vi "SignalReceiver.TestLauncher.vi"() -> ()   [LabVIEW 2020, in "ECU_Diagnose.lvlib" / "SignalReceiver.lvclass"]
doc: "JKI State Machine Objects (SMO) 1.0.0.5\nJKI - JKI\nCopyright (c) 2016, JKI"
uses:
  SignalReceiver.lvclass
  <vilib>/JKI/JKI SMO/SMO/SMO.lvclass
  <vilib>/JKI/JKI SMO/SMO/Typedefs/SMOState --Enum.ctl
  GlobalData_operation.ctl
  C:/Program Files (x86)/National Instruments/LabVIEW 2020/vi.lib/JKI/JKI SMO/SMO/SMO.lvclass
  D:/BingoGithub/ECU_DiagnoseSMO_V001.06/ECU_Diagnose/SignalReceiver/SignalReceiver.lvclass
  Typedefs/Data.ctl
panel:
  out "Waveform Graph":dbl[][](graph)
  out "SignalDatOut":dbl[][](array[numeric])
  in  "StartStop":bool
  out "Value":T1
  in  "Setpoint":dbl(slide) scale=0.0..10.0
  out "error out":errorcluster
  in  "Stop":bool
  # "Timed Loop Test Launcher"
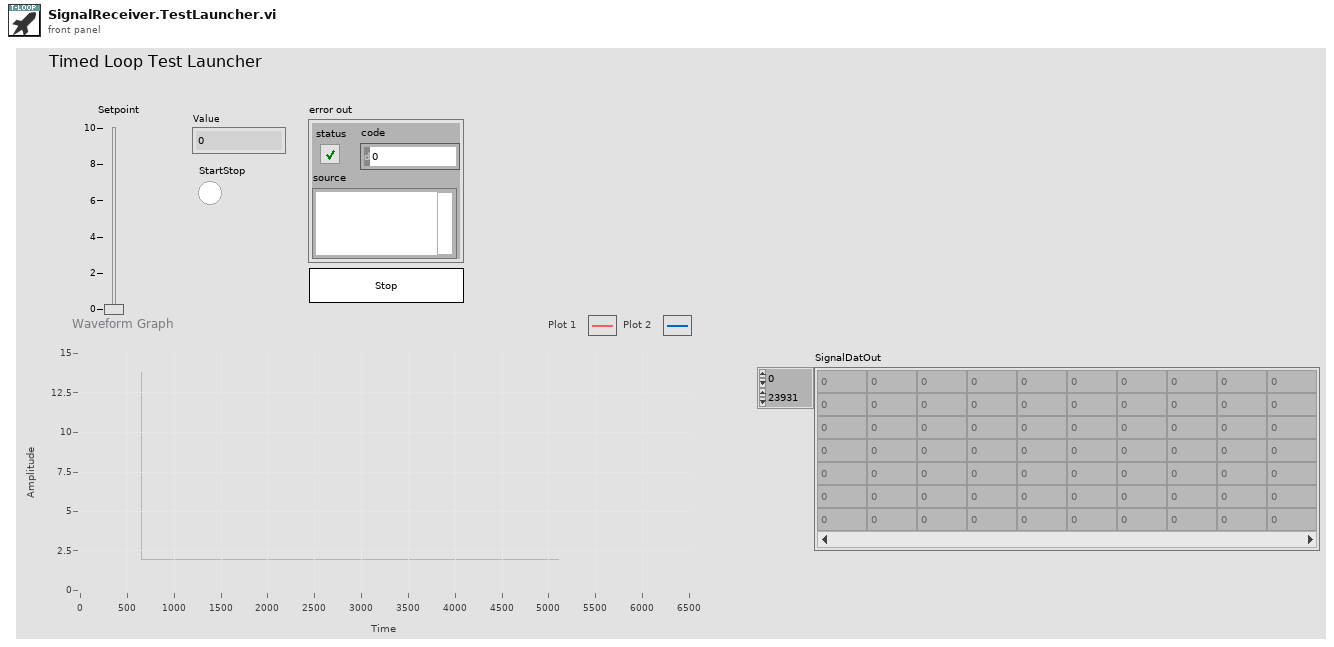
[diagram p1: front panel]
types:
  T1 = typedef "Data.ctl" = dbl
  T2 = typedef "ECU_Diagnose.lvlib/SignalReceiver.lvclass/SignalArrySelecte.ctl" = cluster{"Port_No.":refnum<k21>, "XNET Signal":refnum<k21>[]}
  T3 = typedef "SMO.lvclass/Public Events.ctl" = cluster{"Error":refnum<user-event>, "State":refnum<user-event>, "Reserve State":refnum<user-event>}
  T4 = typedef "ECU_Diagnose.lvlib/SignalReceiver.lvclass/PublicEvents--Cluster.ctl" = cluster{"Setpoint Changed":refnum<user-event>, "Value Changed":refnum<user-event>}
  T5 = typedef "SMO.lvclass/SMOState --Enum.ctl" = enum16{"unknown", "Created", "Started", "Stopped"}
  T6 = typedef "GlobalData_operation.ctl" = enum16{"idle", "read", "write", "clear", "init", "destroy"}
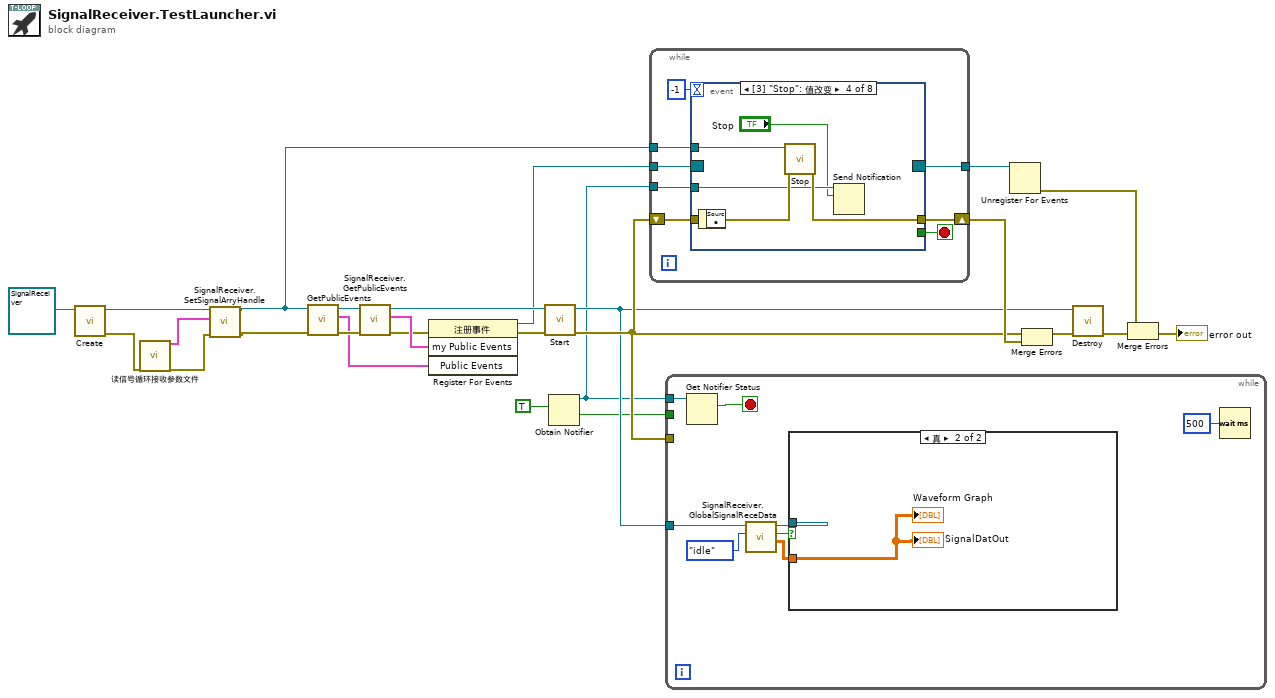
[diagram p0: block diagram]
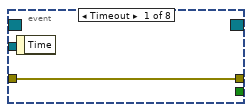
[diagram p3: hidden frame]
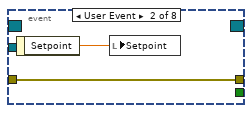
[diagram p4: hidden frame]
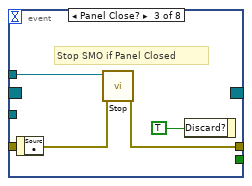
[diagram p5: hidden frame]
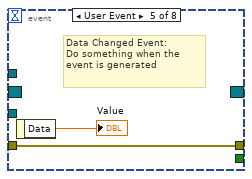
[diagram p6: hidden frame]
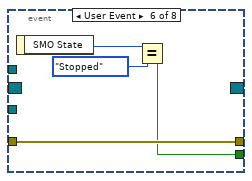
[diagram p7: hidden frame]
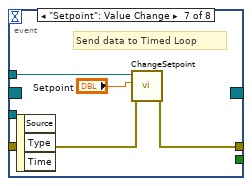
[diagram p8: hidden frame]
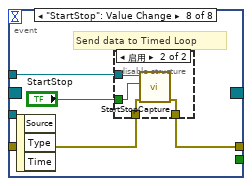
[diagram p9: hidden frame]
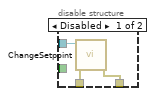
[diagram p10: hidden frame]
diagram:
  n1 = call <vilib>:"Create.vi"("SMO"=refnum<class "SignalReceiver.lvclass"> refnum ("SMO.Template.lvclass")) -> ("error out"=w2:errorcluster, "SMO out"=w11:refnum<class "SignalReceiver.lvclass">)  [unwired: 8 in, 1 out]
  n2 = call "读信号循环接收参数文件.vi"("error in (no error)"=w2) -> ("SignalArryOut"=w1:T2, "error out"=w3:errorcluster)  [unwired: 17 in]
  n3 = call "SignalReceiver.SetSignalArryHandle.vi"("error in (no error)"=w3, "SignalArrySelect"=w1, "SignalReceiver"=w11) -> ("error out"=w9:errorcluster, "SignalReceiver out"=w10:refnum<class "SignalReceiver.lvclass">)  [unwired: 7 in]
  n4 = call <vilib>:"GetPublicEvents.vi"("error in (no error)"=w9, "SMO"=w10) -> ("error out"=w17:errorcluster, "Public Events"=w13:T3, "SMO out"=w16:refnum<class "SignalReceiver.lvclass">)  [unwired: 7 in]
  n5 = call "SignalReceiver.GetPublicEvents.vi"("error in (no error)"=w17, "SignalReceiver"=w16) -> ("error out"=w15:errorcluster, "my Public Events"=w18:T4, "SignalReceiver out"=w19:refnum<class "SignalReceiver.lvclass">)  [unwired: 7 in]
  n6 = register-events(error in=w15, w18, w13) -> (reference out=w12:refnum<event-registration>, error out=w14:errorcluster)  [unwired: 1 in]
  n7 = call <vilib>:"Start.vi"("error in (no error)"=w14, "SMO"=w19) -> ("error out"=w8:errorcluster, "SMO out"=w7:refnum<class "SignalReceiver.lvclass">)  [unwired: 8 in]
  n8 = Obtain Notifier(notification data type=TRUE) -> (notifier out=w4:refnum<notifier>, created new?=w5:bool)  [unwired: 3 in, 1 out]
  n9 = while {
    shift-right: [w33] -> w25
    shift-left: w8 -> [w32]
    tunnel: w12 -> [w31]
    tunnel: [w30] -> w26
    tunnel: w10 -> [w29]
    tunnel: w4 -> [w27]
    stop <- w34 stop-if-true
    n10 = event shown="[3] \"Stop\": 值改变" {
      selector: w31 -> [_ _ _ _ _ _ _ _]
      dyn-events: [_ _ _ _ _ _ _ _] -> w30
      timeout: -1 -> [_ _ _ _ _ _ _ _]
      tunnel: [_ _ _ _ _ w49 _ _] -> w34
      tunnel: w29 -> [_ _ w41 w46 _ _ w56 w60]
      tunnel: [w35 w37 w40 w45 w48 w52 w53 w58] -> w33
      tunnel: w32 -> [w35 w37 w39 w44 w48 w52 w54 w59]
      tunnel: w27 -> [_ _ _ w43 _ _ _ _]
      event Timeout {
        n11 = event-data() -> ()  [unwired: 1 in, 1 out]
      }
      event User Event {
        n12 = event-data() -> ("Setpoint"=w36:T1)  [unwired: 1 in]
        n13 = local write "Setpoint"(w36) -> ()
      }
      event Panel Close? {
        # "Stop SMO if Panel Closed"
        n14 = event-data() -> ()  [unwired: 1 in, 1 out]
        n15 = call <vilib>:"Stop.vi"("error in (no error)"=w39, "SMO"=w41) -> ("error out"=w40:errorcluster)  [unwired: 8 in, 1 out]
        n16 = event-data("Discard?"=TRUE ("OK")) -> ()  [unwired: 1 in, 1 out]
      }
      event "Stop": Value Change {
        n17 = event-data() -> ()  [unwired: 1 in, 1 out]
        n18 = call <vilib>:"Stop.vi"("error in (no error)"=w44, "SMO"=w46) -> ("error out"=w45:errorcluster)  [unwired: 8 in, 1 out]
        n19 = Send Notification(notification="Stop", notifier=w43) -> ()  [unwired: 1 in, 2 out]
      }
      event User Event {
        # "Data Changed Event:\nDo something when the\nevent is generated"
        n20 = event-data() -> ("Data"=→"Value":T1)  [unwired: 1 in]
      }
      event User Event {
        n21 = event-data() -> ("SMO State"=w51:T5)  [unwired: 1 in]
        n22 = Equal?(x=w51, y=SMOState_--Enum."Stopped") -> (x = y?=w49:bool)
      }
      event "Setpoint": Value Change {
        # "Send data to Timed Loop"
        n23 = event-data() -> ()  [unwired: 1 in, 3 out]
        n24 = call "ChangeSetpoint.vi"("error in (no error)"=w54, "Setpoint"="Setpoint", "SignalReceiver"=w56) -> ("error out"=w53:errorcluster)  [unwired: 7 in, 1 out]
      }
      event "StartStop": Value Change {
        # "Send data to Timed Loop"
        n25 = event-data() -> ()  [unwired: 1 in, 3 out]
        n26 = disable-structure shown="启用" {
          disable-tunnel: w60 -> [w63 w67]
          disable-tunnel: w59 -> [w62 w66]
          disable-tunnel: [w61 w65] -> w58
          disable-tunnel: "StartStop" -> [_ w64]
          frame Disabled {
            n27 = call "ChangeSetpoint.vi"("error in (no error)"=w62, "SignalReceiver"=w63) -> ("error out"=w61:errorcluster)  [unwired: 8 in, 1 out]
          }
          frame Enabled {
            n28 = call "StartStopCapture.vi"("error in (no error)"=w66, "StartStopCapture"=w64, "SignalReceiver"=w67) -> ("error out"=w65:errorcluster)  [unwired: 7 in, 1 out]
          }
        }
      }
    }
  }
  n29 = while {
    tunnel: w8 -> [_]
    tunnel: w7 -> [w72]
    tunnel: w5 -> [_]
    tunnel: w4 -> [w70]
    stop <- w69 stop-if-true
    n30 = Get Notifier Status(notifier=w70) -> (current notification=w69:bool)  [unwired: 1 in, 4 out]
    n31 = call "SignalReceiver.GlobalSignalReceData.vi"("operation"=GlobalData_operation."idle", "SignalReceiver"=w72) -> ("SignalDatOut"=w68:dbl[][], "Update"=w73:bool, "SignalReceiver out"=w71:refnum<class "SignalReceiver.lvclass">)  [unwired: 6 in, 1 out]
    n32 = case shown="真" w73 {
      tunnel: w71 -> [_ _]
      tunnel: w68 -> [_ w76]
      frame False {
      }
      frame True {
        "SignalDatOut" <- w76
        "Waveform Graph" <- w76
      }
    }
    n33 = Wait (ms)(milliseconds to wait=u32 500 ("等待时间（毫秒）")) -> ()  [unwired: 1 out]
  }
  n34 = Unregister For Events(event registration refnum=w26) -> (error out=w24:errorcluster)  [unwired: 1 in]
  n35 = Merge Errors(w8, w25) -> (w20:errorcluster)
  n36 = call <vilib>:"Destroy.vi"("error in (no error)"=w20, "SMO"=w7) -> ("error out"=w22:errorcluster)  [unwired: 9 in]
  n37 = Merge Errors(w24, w22) -> (→"error out":errorcluster)
